vi "LED Scroll Main.vi"() -> ()   [LabVIEW 2012]
doc: "This VI demonstrates how to use XControls"
uses:
  XControl/LED Display.xctl
panel:
  in  "Stop Button":bool
  out "LED Display Wired":string(xcontrol)="ABC"
  in  "LED Display Default":string(xcontrol)="NATI +10 "
  # "Overview: This example shows a Scrolling LED sign implemented by an XControl of String data type  and it demonstrates several key ways \nto use an XControls.\nRequirements: LabVIEW 2012 or compatible.\nInstructions:\n1. The first LED XControl will display the default string assigned to it. The second will display the string wired to it. Navigate to the block \n    Diagram to change the value of the string\n2. Run the VI\n3. Right click any of the XContols and click on Set Text from the drop-down menu to change the text being displayed.\n4. Right click any of the XControls and click on Show Diagram to check the code associated to the XControl\n5. You can grow and shrink the XControl. If you grow it in the horizontal, it will add rows to the array, but not if you grow it vertically. \n6. Stop the VI\n7. Run again and notice that the value of the default control was the same from previous run."
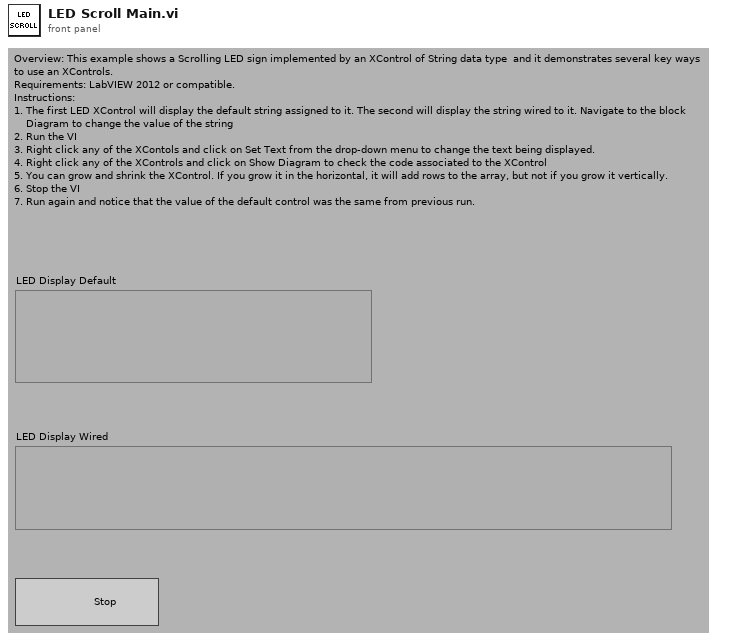
[diagram p1: front panel]
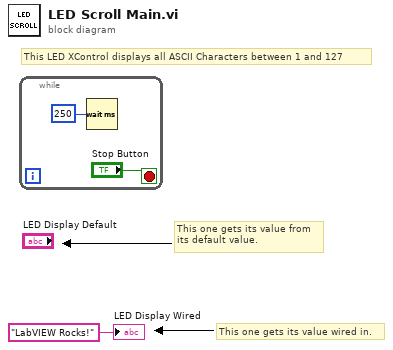
[diagram p0: block diagram]
diagram:
  # "This LED XControl displays all ASCII Characters between 1 and 127"
  # "This one gets its value wired in."
  # "This one gets its value from\nits default value."
  n1 = while {
    stop <- "Stop Button" stop-if-true
    n2 = Wait (ms)(milliseconds to wait=u32 250) -> ()  [unwired: 1 out]
  }
  "LED Display Wired" <- "LabVIEW Rocks!" ("LED Display")
